vi "Global odometry.vi"() -> ()   [LabVIEW 2023]
uses:
  ctrl defs/ctrl driver input.ctl
  ctrl defs/ctrl swerve module.ctl
  ctrl defs/ctrl XY coord.ctl
  <vilib>/Rock Robotics/WPI/DriverStation/WPI_DriverStationAllianceInfo.ctl
  ctrl defs/ctrl DRIVING FRAME selector.ctl
  ctrl defs/ctrl FRONT FACE selector.ctl
  ctrl defs/ctrl LimeLight target.ctl
panel:
  in  "Tab Control":enum32{"Page 1", "Page 2"}(tab)
  in  "Limelight target":T1
  in  "RUN ARMS":T2 {"RIGHT ARM"."VBus%" min=-1.0 max=1.0 step=0.005 format="%#.5f"; "LEFT ARM"."VBus%" min=-1.0 max=1.0 step=0.005 format="%#.5f"}
  in  "front face":T3
  in  "drive frame":T4
  in  "Alliance":T5
  in  "MAGNETIC Zero for Blue Alliance (deg)":dbl=200.5 format="%#.4f"
  in  "pivot center":T6 {"Y" format="%.4g"; "X" format="%.4g"}
  in  "DRIVER INPUT":T7={"Jx"=0.5, "Jy"=-0.5, "Jr "=0.5, "R"=0.7071, "theta (deg)"=45.0, "theta (rad)"=0.785398} {"Jr" format="%.4g"; "theta (rad)" format="%_4f"; "R" format="%.4g"; "Jy" format="%.4g"; "theta (deg)" format="%_4f"; "Jx" format="%.4g"}
  in  "swerve module data":T8[](array[typedef])=[{"descr"="FR", "V"=0.0, "POS"=0.0, "target"=0.0, "ABS"=0.0, "from pivot to module"={"R"=0.0, "theta (deg)"=0.0, "theta spin (deg)"=0.0}, "coord wrt geom CTR"={"X"=12.214, "Y"=12.214}, "corner wt (lbm)"=18.4}, {"descr"="FL", "V"=0.0, "POS"=0.0, "target"=0.0, "ABS"=0.0, "from pivot to module"={"R"=0.0, "theta (deg)"=0.0, "theta spin (deg)"=0.0}, "coord wrt geom CTR"={"X"=-12.214, "Y"=12.214}, "corner wt (lbm)"=16.8}, {"descr"="RL", "V"=0.0, "POS"=0.0, "target"=0.0, "ABS"=0.0, "from pivot to module"={"R"=0.0, "theta (deg)"=0.0, "theta spin (deg)"=0.0}, "coord wrt geom CTR"={"X"=-12.214, "Y"=-12.214}, "corner wt (lbm)"=25.4}, {"descr"="RR", "V"=0.0, "POS"=0.0, "target"=0.0, "ABS"=0.0, "from pivot to module"={"R"=0.0, "theta (deg)"=0.0, "theta spin (deg)"=0.0}, "coord wrt geom CTR"={"X"=12.214, "Y"=-12.214}, "corner wt (lbm)"=22.8}] {"corner wt (lbm)" format="%#.3f"; "POS" format="%.3g"; "coord wrt geom CTR"."Y" format="%.4g"; "coord wrt geom CTR"."X" format="%.4g"; "from pivot to module"."theta spin (deg)" format="%.4g"; "from pivot to module"."theta (deg)" format="%.4g"; "from pivot to module"."R" format="%.4g"; "ABS" format="%.3g"; "target" format="%.3g"; "V" format="%.3g"}
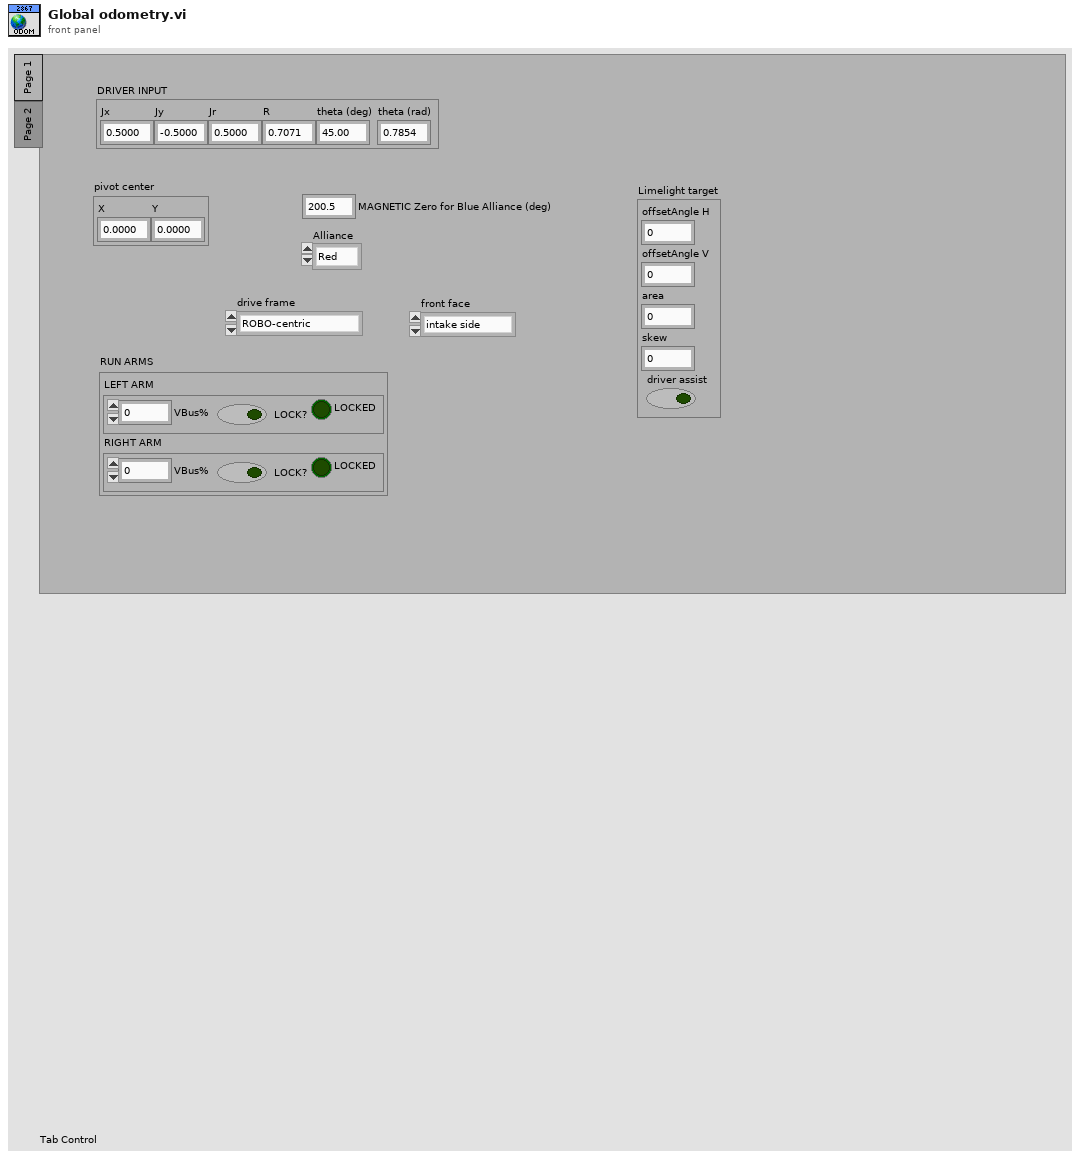
[diagram p1: front panel]
types:
  T1 = typedef "ctrl LimeLight target.ctl" = cluster{"offsetAngle H":dbl, "offsetAngle V":dbl, "area":dbl, "skew":dbl, "driver assist":bool}
  T2 = cluster{"LEFT ARM":cluster{"VBus%":dbl, "LOCK?":bool, "LOCKED":bool}, "RIGHT ARM":cluster{"VBus%":dbl, "LOCK?":bool, "LOCKED":bool}}
  T3 = typedef "ctrl FRONT FACE selector.ctl" = enum16{"intake side", "shooter side"}
  T4 = typedef "ctrl DRIVING FRAME selector.ctl" = enum16{"ROBO-centric", "FLD-centric"}
  T5 = typedef "WPI_DriverStationAllianceInfo.ctl" = enum16{"Red", "Blue", "Invalid"}
  T6 = typedef "ctrl XY coord.ctl" = cluster{"X":dbl, "Y":dbl}
  T7 = typedef "ctrl driver input.ctl" = cluster{"Jx":dbl, "Jy":dbl, "Jr ":dbl, "R":dbl, "theta (deg)":dbl, "theta (rad)":dbl}
  T8 = typedef "ctrl swerve module.ctl" = cluster{"descr":string, "V":dbl, "POS":dbl, "target":dbl, "ABS":dbl, "from pivot to module":cluster{"R":dbl, "theta (deg)":dbl, "theta spin (deg)":dbl}, "coord wrt geom CTR":cluster{"X":dbl, "Y":dbl}, "corner wt (lbm)":dbl}
diagram:
